vi "MainIdent RT.vi"   [LabVIEW 2018]
doc: "The myRIO Project template acquires acceleration data from the onboard accelerometer and displays the changes of acceleration values in a waveform chart."
uses:
  <vilib>/platform/TimedLoop/XDataNode/XDataNode.xnode
  <vilib>/Platform/TimedLoop/XDataNode/nitl_modes.ctl
  <vilib>/Platform/TimedLoop/XDataNode/XDNodeRunTimeDep.lvlib
  <vilib>/Platform/TimedLoop/XDataNode/wakeup.ctl
  <vilib>/Platform/TimedLoop/XDataNode/timing_clust.ctl
  <vilib>/myRIO/Common/Instrument Driver Framework/Utilities/typedefs/Generic FPGA Reference.ctl
  <vilib>/myRIO/Common/Instrument Driver Framework/Utilities/typedefs/myRIO v1.0 Reference.ctl
  <vilib>/myRIO/Common/Instrument Driver Framework/Utilities/typedefs/Hardware Version Enum.ctl
  <vilib>/myRIO/Common/Instrument Driver Framework/Utilities/typedefs/myRIO Generic Hardware Reference.ctl
  <vilib>/userdefined/High Color/nirio_resource_hc.ctl
  <vilib>/myRIO/Common/Instrument Driver Framework/myRIO v1.0/Encoder/typedefs/Encoder Channels Enum.ctl
  <vilib>/myRIO/Instrument Drivers/Onboard IO/Encoder/typedefs/Encoder Reference.ctl
  <vilib>/myRIO/Instrument Drivers/Onboard IO/Encoder/Encoder.lvlib
  <vilib>/myRIO/Common/Instrument Driver Framework/myRIO v1.0/Encoder/typedefs/Encoder Signal Mode.ctl
  <vilib>/myRIO/Instrument Drivers/Onboard IO/Encoder/vis/myRIO Encoder Open.xnode
  <vilib>/myRIO/Common/Instrument Driver Framework/myRIO v1.0/Encoder/vis/myRIO v1.1 Open Encoder.vi
  <vilib>/myRIO/Common/Instrument Driver Framework/myRIO v1.0/Encoder/vis/myRIO v1.0 Configure Encoder.vi
  <vilib>/myRIO/Common/Instrument Driver Framework/myRIO v1.0/Encoder/typedefs/Encoder Configuration v1.0.ctl
  <vilib>/myRIO/Instrument Drivers/Onboard IO/PWM/typedefs/PWM Configuration.ctl
  <vilib>/myRIO/Instrument Drivers/Onboard IO/PWM/PWM.lvlib
  <vilib>/myRIO/Common/Instrument Driver Framework/myRIO v1.0/PWM/typedefs/PWM Channels Enum.ctl
  <vilib>/myRIO/Instrument Drivers/Onboard IO/PWM/typedefs/PWM Reference.ctl
  <vilib>/myRIO/Instrument Drivers/Onboard IO/PWM/vis/myRIO PWM Open.xnode
  <vilib>/myRIO/Common/Instrument Driver Framework/myRIO v1.0/PWM/vis/myRIO v1.1 Open PWM.vi
types:
  T1 = typedef "Encoder Signal Mode.ctl" = enum16{"Quadrature phase signal", "Step and direction signal"}
  T2 = typedef "PWM.lvlib/PWM Reference.ctl" = cluster{"myRIO Reference":T3, "PWM Channels Enum":T7, "PWM Configuration":T8}
  T3 = typedef "myRIO Generic Hardware Reference.ctl" = cluster{"myRIO Model":T4, "myRIO Hardware Reference":T5}
  T4 = typedef "Hardware Version Enum.ctl" = enum16{"Unknown", "myRIO-1900", "myRIO-1950", "roboRIO", "NI ELVIS RIO CM", "ELVIS III"}
  T5 = typedef "myRIO v1.0 Reference.ctl" = cluster{"Generic FPGA Reference":T6, "Allow multiple opens":bool}
  T6 = typedef "Generic FPGA Reference.ctl" = refnum<k20>
  T7 = typedef "PWM Channels Enum.ctl" = enum16{"Not Connected", "C/PWM0", "C/PWM1", "A/PWM0", "A/PWM1", "A/PWM2", "A/PWM3", "A/PWM4", "A/PWM5", "A/PWM6", "A/PWM7", "A/PWM8", "A/PWM9", "A/PWM10", "A/PWM11", "A/PWM12", "A/PWM13", "A/PWM14", "A/PWM15", "A/PWM16", "A/PWM17", "A/PWM18", "A/PWM19", "B/PWM0", "B/PWM1", "B/PWM2", "B/PWM3", "B/PWM4", "B/PWM5", "B/PWM6", "B/PWM7", "B/PWM8", "B/PWM9", "B/PWM10", "B/PWM11", "B/PWM12", "B/PWM13", "B/PWM14", "B/PWM15", "B/PWM16", "B/PWM17", "B/PWM18", "B/PWM19", "PWM/PWM0", "PWM/PWM1", "PWM/PWM2", "PWM/PWM3", "PWM/PWM4", "PWM/PWM5", "PWM/PWM6", "PWM/PWM7", "PWM/PWM8", "PWM/PWM9"}
  T8 = typedef "PWM.lvlib/PWM Configuration.ctl" = cluster{"Frequency":dbl, "Duty Cycle":dbl}
  T9 = typedef "Encoder.lvlib/Encoder Reference.ctl" = cluster{"myRIO Reference":T3, "Encoder Channels Enum":T10}
  T10 = typedef "Encoder Channels Enum.ctl" = enum16{"Not Connected", "C/ENC0", "C/ENC1", "A/ENC", "A/ENC0", "A/ENC1", "A/ENC2", "A/ENC3", "A/ENC4", "A/ENC5", "A/ENC6", "A/ENC7", "A/ENC8", "A/ENC9", "B/ENC", "B/ENC0", "B/ENC1", "B/ENC2", "B/ENC3", "B/ENC4", "B/ENC5", "B/ENC6", "B/ENC7", "B/ENC8", "B/ENC9", "DIO/ENC0", "DIO/ENC1", "DIO/ENC2", "DIO/ENC3", "DIO/ENC4"}
  T11 = typedef "XDNodeRunTimeDep.lvlib/timing_clust.ctl" = cluster{"Expected End [f-1]":u64, "Actual End [f-1]":u64, "Finished Late? [f-1]":bool, "Expected End [i-1]":u64, "Actual End [i-1]":u64, "Finished Late? [i-1]":bool, "Expected Start [i]":u64, "Actual Start [i]":u64, "Expected Start [f]":u64, "Actual Start [f]":u64, "Source Name":string, "Structure Name":string, "Period":i64, "Deadline":i64, "Offset":i64, "Start":i64, "Priority":i32, "Timeout":i32, "Mode":T12, "Wakeup Reason":T13, "Error":errorcluster, "Source Type":string, "Secondary Source Type":string, "Global End Time":u64, "Global Start Time":u64, "Frame Duration":u64, "Iteration Duration":u64, "Assigned CPU":i32, "I/O Scan Engine Mode":u32}
  T12 = typedef "XDNodeRunTimeDep.lvlib/nitl_modes.ctl" = enum32{"No Change", "Process missed periods, maintain original phase", "Discard missed periods, maintain original phase", "Process missed periods, ignore original phase", "Discard missed periods, ignore original phase"}
  T13 = typedef "XDNodeRunTimeDep.lvlib/wakeup.ctl" = enum32{"Normal", "Aborted", "Asynchronous wakeup", "Timing source error", "Timed loop error", "Timeout"}
  T14 = cluster{"Double":dbl, dbl, "Double":dbl, "seconds since 1Jan1904":timestamp}
  T15 = cluster{"Double":dbl, "dbl Scaled Value":dbl, "Output":dbl, "seconds since 1Jan1904":timestamp}
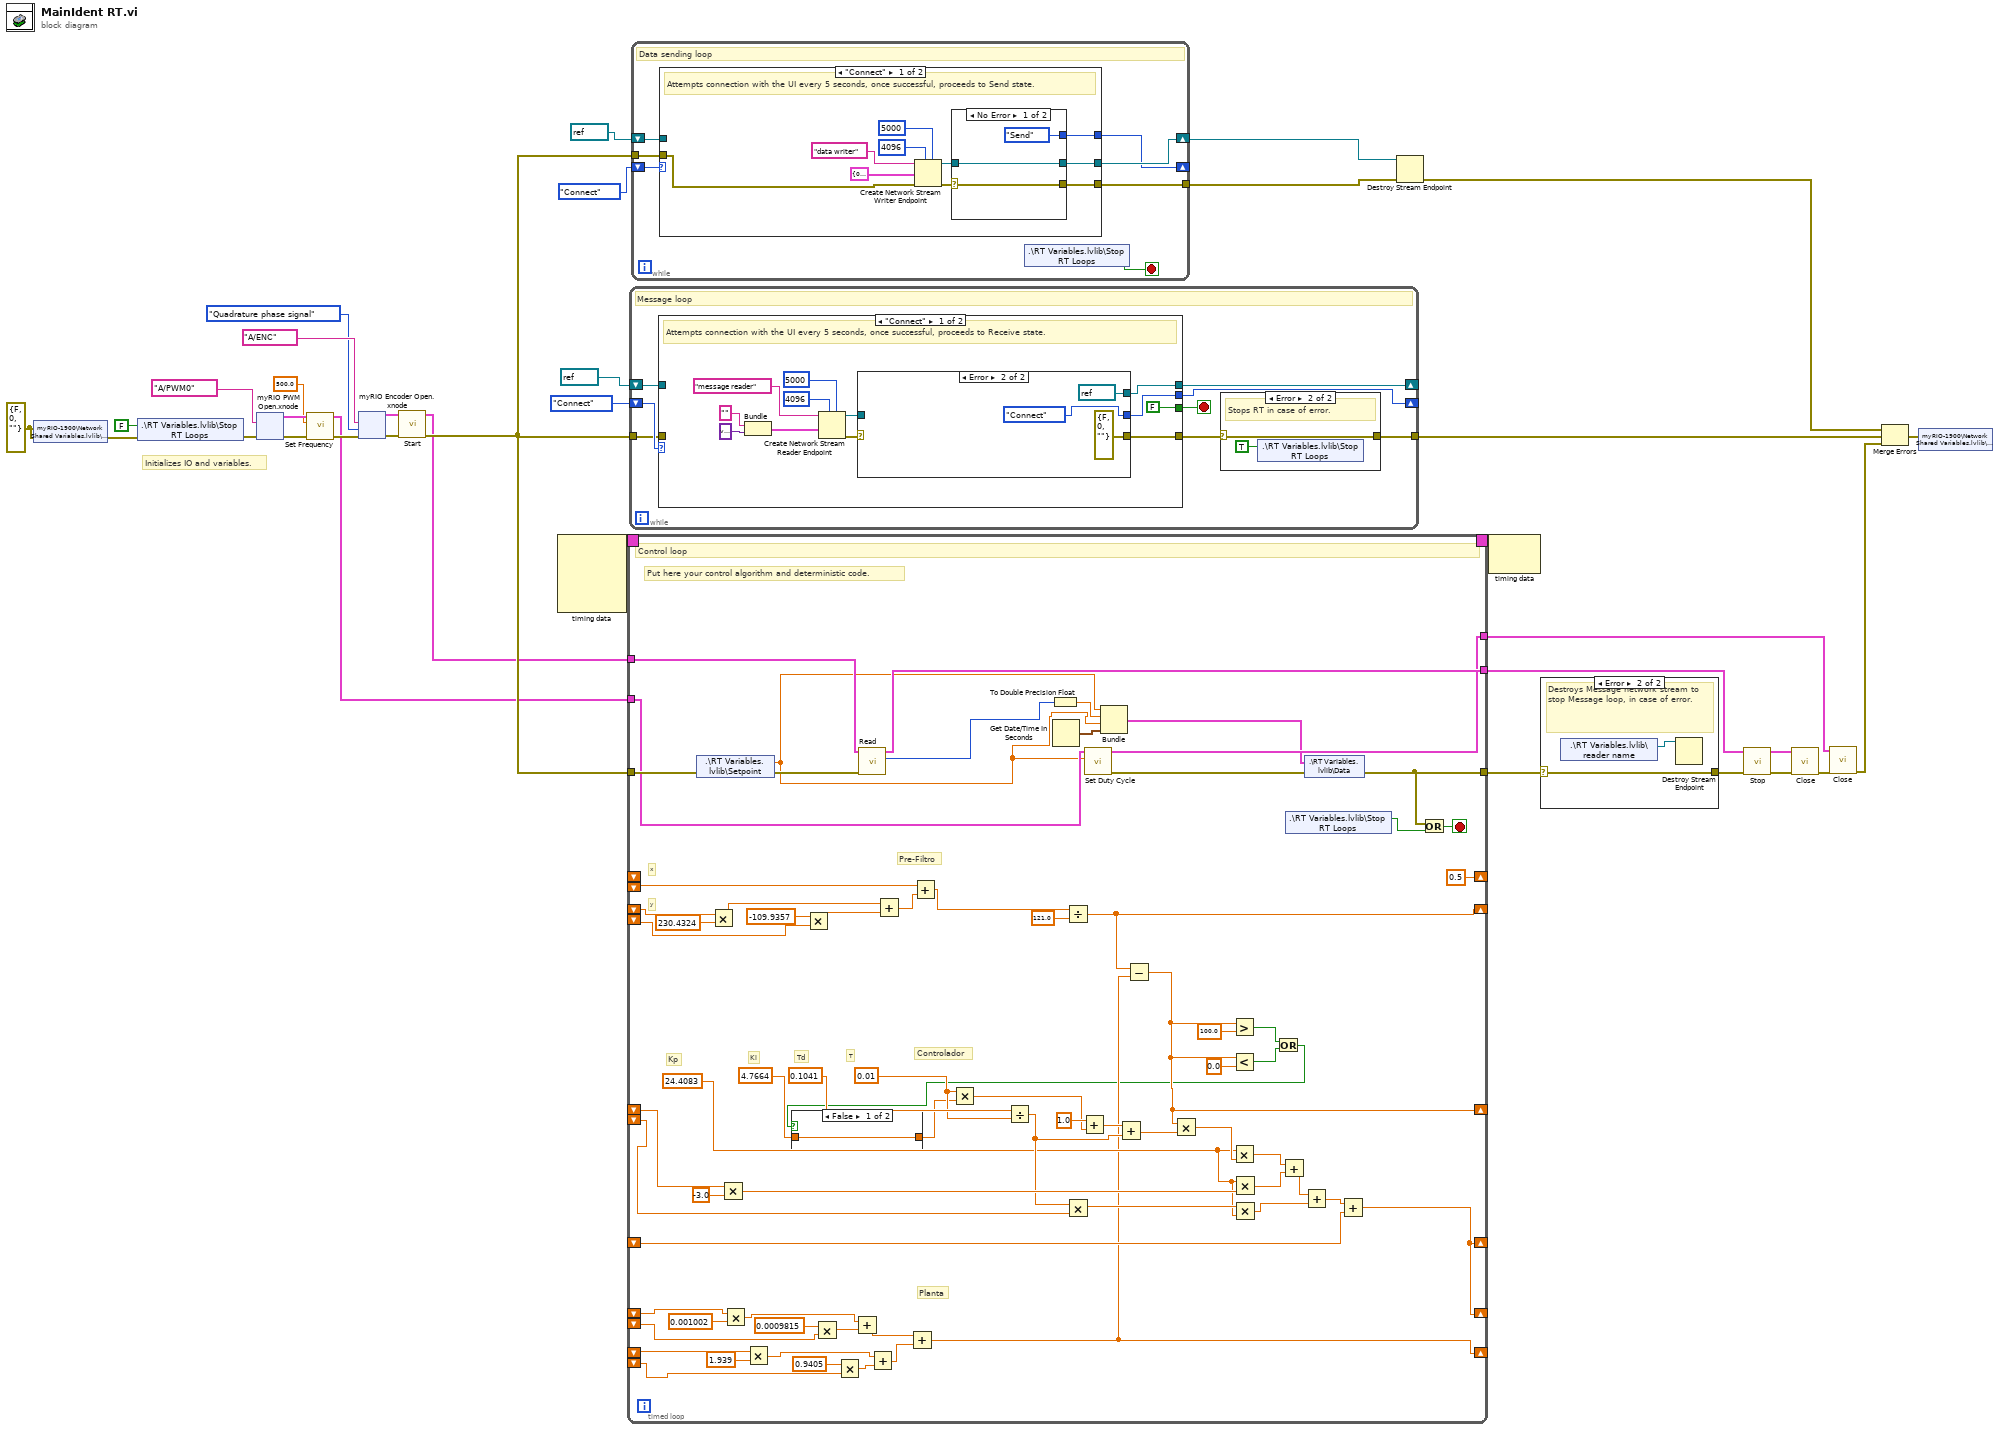
[diagram p0: block diagram]
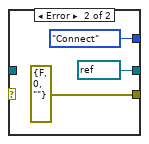
[diagram p3: hidden frame]
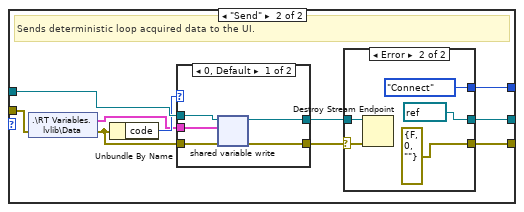
[diagram p4: hidden frame]
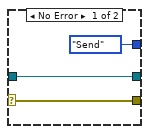
[diagram p5: hidden frame]
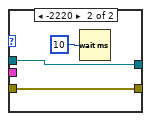
[diagram p6: hidden frame]
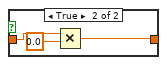
[diagram p7: hidden frame]
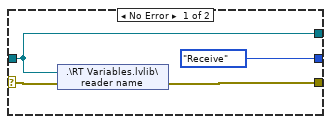
[diagram p9: hidden frame]
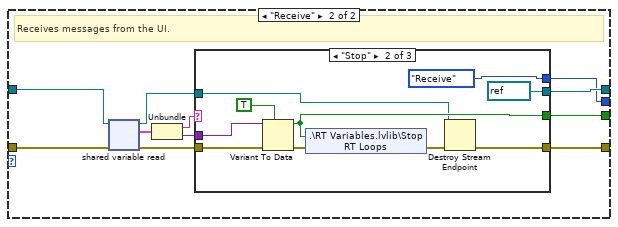
[diagram p10: hidden frame]
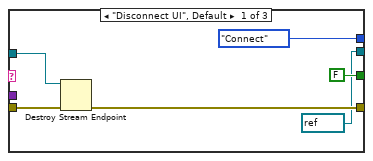
[diagram p11: hidden frame]
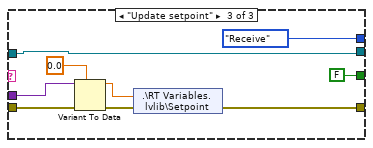
[diagram p12: hidden frame]
diagram:
  w22 = errorcluster {"status"=FALSE, "code"=0, "source"=""} ("error IO")
  # "Initializes IO and variables."
  n1 = shared-variable "myRIO-1900\\Network Shared Variables.lvlib\\error IO"(w22, error in=w22) -> (error out=w23:errorcluster)
  n2 = shared-variable ".\\RT Variables.lvlib\\Stop RT Loops"(FALSE ("Stop RT Loops"), error in=w23) -> (error out=w8:errorcluster)
  n3 = xnode "myRIO PWM Open.xnode"("error in (no error)"=w8, "Channel Name"=tag "A/PWM0") -> ("error out"=w10:errorcluster, "PWM Ref Out"=w9:T2)  [unwired: 1 in]
  n4 = call <vilib>:"Set Frequency.vi"("error in (no error)"=w10, "Frequency [Hz]"=500.0, "PWM Ref In"=w9) -> ("error out"=w7:errorcluster, "PWM Ref Out"=w4:T2)  [unwired: 6 in]
  n5 = xnode "myRIO Encoder Open.xnode"("error in (no error)"=w7, "Channel Name"=tag "A/ENC", "Encoder Signal Mode"=Encoder_Signal_Mode."Quadrature phase signal") -> ("error out"=w19:errorcluster, "Encoder Ref Out"=w18:T9)  [unwired: 2 in]
  n6 = call <vilib>:"Start.vi"("error in (no error)"=w19, "Encoder Ref In"=w18) -> ("error out"=w16:errorcluster, "Encoder Ref Out"=w15:T9)  [unwired: 8 in]
  n7 = node-c288() -> (w35:T11)  [unwired: 4 in]
  n8 = timed-loop {
    timing: w35 -> [_]
    timing-out: [_] -> w34
    tunnel: w16 -> [w105]
    tunnel: [w101] -> w21
    tunnel: w15 -> [w100]
    tunnel: [w99] -> w11
    tunnel: w4 -> [w97]
    tunnel: [w94] -> w3
    shift-right: [0.5] -> _
    shift-left: _ -> [_]
    shift-right: [w44] -> _
    shift-left: _ -> [w90]
    shift-left: _ -> [w84]
    shift-left: _ -> [w89]
    shift-right: [w40] -> _
    shift-left: _ -> [w60]
    shift-right: [w46] -> _
    shift-left: _ -> [w49]
    shift-left: _ -> [w57]
    shift-right: [w46] -> _
    shift-left: _ -> [w48]
    shift-right: [w45] -> _
    shift-left: _ -> [w76]
    shift-left: _ -> [w47]
    shift-left: _ -> [w75]
    stop <- w102 stop-if-true
    w64 = 0.01
    w55 = 24.4083
    # "Planta"
    # "Controlador"
    # "Pre-Filtro"
    # "T"
    # "Td"
    # "Ki"
    # "Kp"
    # "y"
    # "x"
    # "Put here your control algorithm and deterministic code."
    # "Control loop"
    n9 = shared-variable ".\\RT Variables.lvlib\\Setpoint"(error in=w105) -> (w92:dbl, error out=w106:errorcluster)
    n10 = Multiply(x=w90, y=230.4324) -> (x*y=w87:dbl)
    n11 = Multiply(x=w60, y=-3.0) -> (x*y=w59:dbl)
    n12 = Multiply(x=w48, y=0.001002) -> (x*y=w74:dbl)
    n13 = Multiply(x=w76, y=1.939) -> (x*y=w71:dbl)
    n14 = Multiply(x=-109.9357, y=w89) -> (x*y=w86:dbl)
    n15 = Multiply(x=0.0009815, y=w47) -> (x*y=w73:dbl)
    n16 = Multiply(x=0.9405, y=w75) -> (x*y=w72:dbl)
    n17 = Add(x=w74, y=w73) -> (x+y=w69:dbl)
    n18 = call <vilib>:"Read.vi"("error in (no error)"=w106, "Encoder Ref In"=w100) -> ("Counter Value"=w96:i32, "Encoder Ref Out"=w99:T9)  [unwired: 5 in, 3 out]
    n19 = Add(x=w71, y=w72) -> (x+y=w70:dbl)
    n20 = Add(x=w87, y=w86) -> (x+y=w85:dbl)
    n21 = Add(x=w69, y=w70) -> (x+y=w45:dbl)
    n22 = Add(x=w84, y=w85) -> (x+y=w82:dbl)
    n23 = Divide(x=0.1041, y=w64) -> (x/y=w58:dbl)
    n24 = To Double Precision Float(number=w96) -> (double precision float=w95:dbl)
    n25 = Get Date/Time In Seconds() -> (seconds since 1Jan1904=w104:timestamp)
    n26 = Divide(x=w82, y=121.0) -> (x/y=w44:dbl)
    n27 = Multiply(x=w58, y=w57) -> (x*y=w56:dbl)
    n28 = call <vilib>:"Set Duty Cycle.vi"("Duty Cycle"=w92, "PWM Ref In"=w97) -> ("error out"=w98:errorcluster, "PWM Ref Out"=w94:T2)  [unwired: 7 in]
    n29 = Bundle("Double"=w92, w95, "Double"=w92, "seconds since 1Jan1904"=w104) -> (w93:T14)  [unwired: 1 in]
    n30 = Subtract(x=w44, y=w45) -> (x-y=w40:dbl)
    n31 = Greater?(x=w40, y=100.0) -> (0:w38:bool)
    n32 = Less?(x=w40, y=0.0) -> (x < y?=w37:bool)
    n33 = Multiply(x=w55, y=w59) -> (x*y=w53:dbl)
    n34 = Multiply(x=w56, y=w55) -> (x*y=w51:dbl)
    n35 = Or(x=w38, y=w37) -> (x .or. y?=w36:bool)
    n36 = case shown="False" w36 {
      tunnel: 4.7664 -> [w107 w110]
      tunnel: [w107 w108] -> w42
      frame False {
      }
      frame True {
        n37 = Multiply(x=w110, y=0.0) -> (x*y=w108:dbl)
      }
    }
    n38 = Multiply(x=w64, y=w42) -> (x*y=w67:dbl)
    n39 = Add(x=1.0, y=w67) -> (x+y=w66:dbl)
    n40 = Add(x=w66, y=w58) -> (x+y=w63:dbl)
    n41 = Multiply(x=w40, y=w63) -> (x*y=w62:dbl)
    n42 = Multiply(x=w55, y=w62) -> (x*y=w54:dbl)
    n43 = Add(x=w54, y=w53) -> (x+y=w52:dbl)
    n44 = shared-variable ".\\RT Variables.lvlib\\Stop RT Loops"() -> (w103:bool)  [unwired: 1 in, 1 out]
    n45 = Add(x=w52, y=w51) -> (x+y=w50:dbl)
    n46 = shared-variable ".\\RT Variables.lvlib\\Data"(w93, error in=w98) -> (error out=w101:errorcluster)
    n47 = Add(x=w50, y=w49) -> (x+y=w46:dbl)
    n48 = Or(x=w101, y=w103) -> (x .or. y?=w102:bool)
  }
  n49 = while {
    tunnel: [w113] -> w25
    shift-right: [w119] -> _
    shift-left: refnum<k21> refnum ("reader name") -> [w117]
    shift-right: [w118] -> _
    shift-left: enum16{"Connect", "Receive"}."Connect" ("Message states") -> [w120]
    tunnel: w16 -> [w115]
    stop <- w116 stop-if-true
    # "Message loop"
    n50 = case shown="\"Connect\"" w120 {
      tunnel: [w126 w146] -> w114
      tunnel: [w125 w148] -> w119
      tunnel: [w133 w143] -> w118
      tunnel: w117 -> [_ w153]
      tunnel: w115 -> [_ w145]
      tunnel: [FALSE ("Stop RT Loops") w144] -> w116
      frame "Connect" {
        # "Attempts connection with the UI every 5 seconds, once successful, proceeds to Receive state."
        n51 = Bundle("", variant) -> (w129:cluster{string, variant})  [unwired: 1 in]
        n52 = Create Network Stream Reader Endpoint(5:5000 ("timeout in ms (-1)"), 7:4096 ("reader buffer size"), 9:w129, 11:"message reader" ("reader name")) -> (0:w128:errorcluster, 3:w124:refnum<k21>)  [unwired: 3 in]
        n53 = case shown="Error" w128 {
          selector: w128 -> [w137 _]
          tunnel: [enum16{"Connect", "Receive"}."Receive" ("Message states") enum16{"Connect", "Receive"}."Connect" ("Message states")] -> w133
          tunnel: [w136 errorcluster {"status"=FALSE, "code"=0, "source"=""} ("error IO")] -> w126
          tunnel: [w138 refnum<k21> refnum ("reader name")] -> w125
          tunnel: w124 -> [w138 _]
          frame No Error {
            n54 = shared-variable ".\\RT Variables.lvlib\\reader name"(w138, error in=w137) -> (error out=w136:errorcluster)
          }
          frame Error {
          }
        }
      }
      frame "Receive" {
        # "Receives messages from the UI."
        n55 = shared-variable-read(w153, w145) -> (w147:refnum<k21>, w149:errorcluster, w152:cluster{string, variant})  [unwired: 1 in, 1 out]
        n56 = Unbundle(w152) -> (w151:string, w150:variant)
        n57 = case shown="\"Stop\"" w151 {
          tunnel: w150 -> [_ w167 w178]
          tunnel: w149 -> [w157 w169 w177]
          tunnel: [w156 w163 w173] -> w146
          tunnel: [refnum<k21> refnum ("reader name") refnum<k21> refnum ("reader name") w172] -> w148
          tunnel: w147 -> [w155 w162 w172]
          tunnel: [FALSE ("Stop RT Loops") w166 FALSE ("Stop RT Loops")] -> w144
          tunnel: [enum16{"Connect", "Receive"}."Connect" ("Message states") enum16{"Connect", "Receive"}."Receive" ("Message states") enum16{"Connect", "Receive"}."Receive" ("Message states")] -> w143
          frame "Disconnect UI", Default {
            n58 = Destroy Stream Endpoint(8:w157, 11:w155) -> (0:w156:errorcluster)
          }
          frame "Stop" {
            n59 = Variant To Data(error in=w169, type=TRUE ("Stop RT Loops"), Variant=w167) -> (data=w166:bool, error out=w168:errorcluster)
            n60 = shared-variable ".\\RT Variables.lvlib\\Stop RT Loops"(w166, error in=w168) -> (error out=w164:errorcluster)
            n61 = Destroy Stream Endpoint(8:w164, 11:w162) -> (0:w163:errorcluster)
          }
          frame "Update setpoint" {
            n62 = Variant To Data(error in=w177, type=0.0, Variant=w178) -> (data=w175:dbl, error out=w174:errorcluster)
            n63 = shared-variable ".\\RT Variables.lvlib\\Setpoint"(w175, error in=w174) -> (error out=w173:errorcluster)
          }
        }
      }
    }
    n64 = case shown="Error" w114 {
      selector: w114 -> [w121 w122]
      tunnel: [w121 w122] -> w113
      frame No Error {
        # "No action required."
      }
      frame Error {
        # "Stops RT in case of error."
        n65 = shared-variable ".\\RT Variables.lvlib\\Stop RT Loops"(TRUE ("Stop RT Loops")) -> ()  [unwired: 1 in, 1 out]
      }
    }
  }
  n66 = while {
    shift-right: [w183] -> w28
    shift-left: refnum<k21> refnum ("writer endpoint") -> [w181]
    tunnel: [w182] -> w29
    tunnel: w16 -> [w180]
    shift-right: [w179] -> _
    shift-left: enum16{"Connect", "Send"}."Connect" ("Message states") -> [w184]
    stop <- w185 stop-if-true
    # "Data sending loop"
    n67 = case shown="\"Connect\"" w184 {
      tunnel: [w188 w204] -> w182
      tunnel: [w186 w202] -> w183
      tunnel: [w193 w205] -> w179
      tunnel: w181 -> [_ w211]
      tunnel: w180 -> [w189 w210]
      frame "Connect" {
        # "Attempts connection with the UI every 5 seconds, once successful, proceeds to Send state."
        n68 = Create Network Stream Writer Endpoint(5:5000 ("timeout in ms (-1)"), 7:4096 ("writer buffer size"), 8:w189, 9:T15 {"Double"=0.0, "dbl Scaled Value"=0.0, "Output"=0.0, "seconds since 1Jan1904"=timestamp(0 s since 1904-01-01)} ("Data"), 11:"data writer" ("writer name")) -> (0:w191:errorcluster, 3:w187:refnum<k21>)  [unwired: 2 in]
        n69 = case shown="No Error" w191 {
          selector: w191 -> [w196 _]
          tunnel: [enum16{"Connect", "Send"}."Send" ("Message states") enum16{"Connect", "Send"}."Connect" ("Message states")] -> w193
          tunnel: [w196 errorcluster {"status"=FALSE, "code"=0, "source"=""} ("error IO")] -> w188
          tunnel: w187 -> [w198 _]
          tunnel: [w198 refnum<k21> refnum ("writer endpoint")] -> w186
          frame No Error {
          }
          frame Error {
          }
        }
      }
      frame "Send" {
        # "Sends deterministic loop acquired data to the UI."
        n70 = shared-variable ".\\RT Variables.lvlib\\Data"(error in=w210) -> (w207:T15, error out=w209:errorcluster)
        n71 = Unbundle By Name(w209) -> ("code"=w208:i32)
        n72 = case shown="0, Default" w208 {
          tunnel: [w224 w226] -> w206
          tunnel: [w223 w225] -> w203
          tunnel: w211 -> [w222 w225]
          tunnel: w209 -> [w221 w226]
          tunnel: w207 -> [w220 _]
          frame 0, Default {
            n73 = shared-variable-write(w222, w221, w220) -> (w223:refnum<k21>, w224:errorcluster)  [unwired: 1 in, 1 out]
          }
          frame -2220 {
            n74 = Wait (ms)(milliseconds to wait=u32 10) -> ()  [unwired: 1 out]
          }
        }
        n75 = case shown="Error" w206 {
          selector: w206 -> [w214 w218]
          tunnel: [enum16{"Connect", "Send"}."Send" ("Message states") enum16{"Connect", "Send"}."Connect" ("Message states")] -> w205
          tunnel: [w214 errorcluster {"status"=FALSE, "code"=0, "source"=""} ("error IO")] -> w204
          tunnel: w203 -> [w212 w217]
          tunnel: [w212 refnum<k21> refnum ("writer endpoint")] -> w202
          frame No Error {
          }
          frame Error {
            n76 = Destroy Stream Endpoint(8:w218, 11:w217) -> ()  [unwired: 1 out]
          }
        }
      }
    }
    n77 = shared-variable ".\\RT Variables.lvlib\\Stop RT Loops"() -> (w185:bool)  [unwired: 1 in, 1 out]
  }
  n78 = Destroy Stream Endpoint(8:w29, 11:w28) -> (0:w26:errorcluster)
  n79 = node-c288(w34) -> ()  [unwired: 1 out]
  n80 = case shown="Error" w21 {
    selector: w21 -> [w228 w229]
    tunnel: [w228 w229] -> w12
    frame No Error {
      # "No action required."
    }
    frame Error {
      # "Destroys Message network stream to stop Message loop, in case of error."
      n81 = shared-variable ".\\RT Variables.lvlib\\reader name"() -> (w230:refnum<k21>)  [unwired: 1 in, 1 out]
      n82 = Destroy Stream Endpoint(11:w230) -> ()  [unwired: 1 in, 1 out]
    }
  }
  n83 = call <vilib>:"Stop.vi"("error in (no error)"=w12, "Encoder Ref In"=w11) -> ("error out"=w13:errorcluster, "Encoder Ref Out"=w14:T9)  [unwired: 8 in]
  n84 = call <vilib>:"Close.vi"("error in (no error)"=w13, "Encoder Ref In"=w14) -> ("error out"=w6:errorcluster)  [unwired: 9 in]
  n85 = call <vilib>:"Close.vi"("error in (no error)"=w6, "PWM Ref In"=w3) -> ("error out"=w5:errorcluster)  [unwired: 9 in]
  n86 = Merge Errors(w26, w25, w5) -> (w24:errorcluster)
  n87 = shared-variable "myRIO-1900\\Network Shared Variables.lvlib\\error IO"(w24) -> ()  [unwired: 1 in, 1 out]
